vi "Write Record Data.vi"(8 "Error In (no error)":errorcluster, 10 "Record":variant, 11 "Expenses Tracker Saving Goal In":refnum<class "Expenses Tracker Saving Goal.lvclass">) -> (0 "Error Out":errorcluster, 3 "Expenses Tracker Saving Goal Out":refnum<class "Expenses Tracker Saving Goal.lvclass">)   [LabVIEW 2023, in "Expenses Tracker Saving Goal.lvclass"]
uses:
  Expenses Tracker Saving Goal.lvclass
  Expenses Tracker Record/Public/Ctrls/Saving Goal.ctl
  Expenses Tracker Saving Goal.lvclass/Expenses Tracker Saving Goal.ctl
  Expenses Tracker Record/Expenses Tracker Record.lvclass
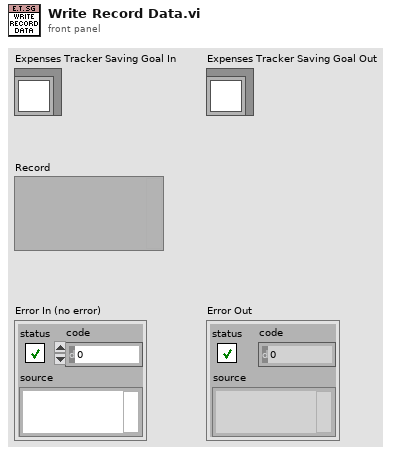
[diagram p1: front panel]
types:
  T1 = typedef "Expenses Tracker Record.lvclass/Saving Goal.ctl" = cluster{"ID":u32, "Name":string, "Current_value":dbl, "Target_value":dbl, "Date_of_entry":timestamp, "Due_date":timestamp, "Last_update":timestamp, "Description":string}
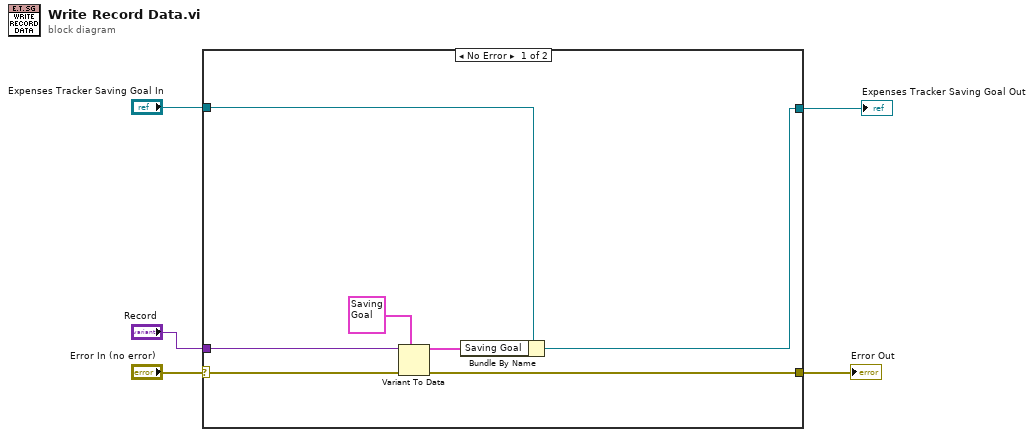
[diagram p0: block diagram]
diagram:
  n1 = case shown="No Error" "Error In (no error)" {
    selector: "Error In (no error)" -> [w10 w14]
    tunnel: [w8 w14] -> w4
    tunnel: [w7 w13] -> w3
    tunnel: "Expenses Tracker Saving Goal In" -> [w6 w13]
    tunnel: "Record" -> [w12 _]
    frame No Error {
      n2 = Variant To Data(error in=w10, type=T1 {"ID"=0, "Name"="", "Current_value"=0.0, "Target_value"=0.0, "Date_of_entry"=timestamp(0 s since 1904-01-01), "Due_date"=timestamp(0 s since 1904-01-01), "Last_update"=timestamp(0 s since 1904-01-01), "Description"=""} ("Saving Goal"), Variant=w12) -> (data=w11:T1, error out=w8:errorcluster)
      n3 = Bundle By Name(cluster=w6, "Saving Goal"=w11) -> (w7:refnum<class "Expenses Tracker Saving Goal.lvclass">)
    }
    frame Error {
    }
  }
  "Error Out" <- w4
  "Expenses Tracker Saving Goal Out" <- w3
